vi "Parse_tags.vi"(10 "XPath expression":string, 11 "XML":string) -> (3 "String":i32)   [LabVIEW 2015]
panel:
  out "Search Results":string[](array[string])
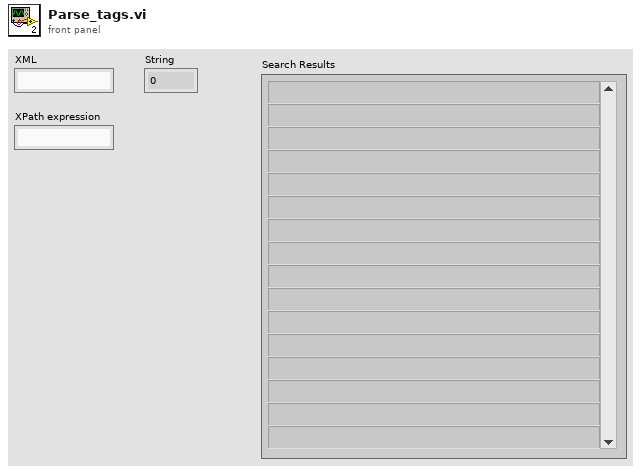
[diagram p1: front panel]
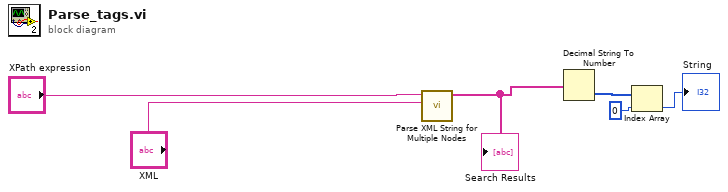
[diagram p0: block diagram]
diagram:
  n1 = call "Parse XML String for Multiple Nodes.vi"("XML String"="XML", "XPath Expression"="XPath expression") -> ("Search Results"=w6:string[])  [unwired: 9 in]
  "Search Results" <- w6
  n2 = Decimal String To Number(string=w6) -> (number=w4:i32[])  [unwired: 2 in, 1 out]
  n3 = Index Array(array=w4, index=0) -> (element=→"String":i32)
